vi "wait.vi"(0 "HGF_Event":refnum<class "HGF_Event.lvclass">, 3 "msTimeout (-1)":i32=-1, 5 "error in (no error)":errorcluster, 9 "ignore previous (F)":bool) -> (14 "dup HGF_Event":refnum<class "HGF_Event.lvclass">, 16 "Object":refnum<class>, 17 "timed out":bool, 19 "error out":errorcluster)   [LabVIEW 2014, in "HGF_BaseClasses.lvlib" / "HGF_Event.lvclass"]
doc: "Use this VI to wait on events.\n\n<b>Hint:</b> This is a shared reentrant VI."
uses:
  HGF_Event.lvclass
  HGF_Auxiliary/HGF_Auxiliary.lvlib
  HGF_Auxiliary/ErrorCode.ctl
  HGF_Auxiliary/Severity.ctl
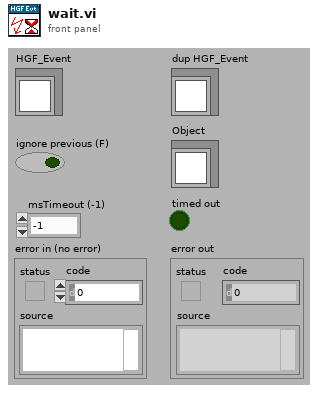
[diagram p1: front panel]
types:
  T1 = typedef "HGF_Auxiliary.lvlib/Severity.ctl" = enum16{"Info", "Warning", "Fault", "Error", "Fatal"}
  T2 = typedef "HGF_Auxiliary.lvlib/ErrorCode.ctl" = enum32{"No error", "Function not supported.", "This VI is for friends only.", "Reference object aready exisits.", "Parameter out of range.", "Not a rendezvous.", "Invalid notifier reference.", "Invalid queue reference.", "Self-Test not supported.", "Reset not supported.", "IDN query not supported.", "Error query not supported.", "Incorrect addressee.", "Object already exists.", "No class name specified", "Driver not supported", "Attribute is not writable"}
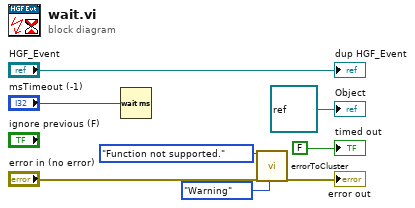
[diagram p0: block diagram]
diagram:
  n1 = Wait (ms)(milliseconds to wait="msTimeout (-1)") -> ()  [unwired: 1 out]
  n2 = call "errorToCluster.vi"("error code"=ErrorCode."Function not supported.", "error in (no error)"="error in (no error)", "severity (Error)"=Severity."Warning") -> ("error out"=→"error out":errorcluster)  [unwired: 2 in, 14 out]
  "dup HGF_Event" <- "HGF_Event"
  "timed out" <- FALSE ("timed out")
  "Object" <- refnum<class> refnum ("Object")
